vi "GLOBAL CHECKER (PC).vi"() -> ()   [LabVIEW 2013]
panel:
  out "Double 2":dbl
  out "Double 1":dbl
  out "Error 2":bool
  out "Error 1":bool
  # "0.00875"
  # "FF_m of speed controlled by CMD"
  # "-2.5"
  # "FF_b of speed controlled by CMD"
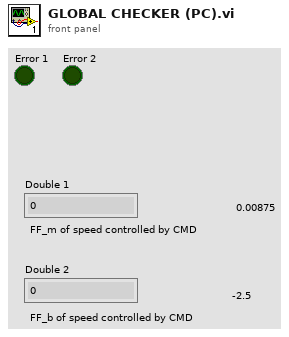
[diagram p1: front panel]
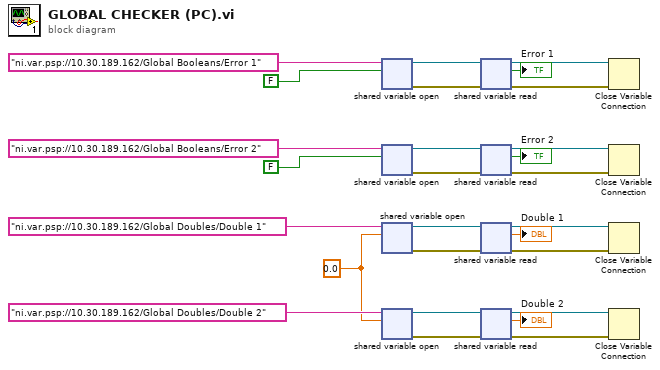
[diagram p0: block diagram]
diagram:
  w3 = 0.0
  n1 = shared-variable-open("ni.var.psp://10.30.189.162/Global Booleans/Error 1", FALSE) -> (w25:refnum<k21>, w22:errorcluster)  [unwired: 2 in]
  n2 = shared-variable-open("ni.var.psp://10.30.189.162/Global Booleans/Error 2", FALSE) -> (w18:refnum<k21>, w21:errorcluster)  [unwired: 2 in]
  n3 = shared-variable-open("ni.var.psp://10.30.189.162/Global Doubles/Double 1", w3) -> (w5:refnum<k21>, w8:errorcluster)  [unwired: 2 in]
  n4 = shared-variable-open("ni.var.psp://10.30.189.162/Global Doubles/Double 2", w3) -> (w12:refnum<k21>, w9:errorcluster)  [unwired: 2 in]
  n5 = shared-variable-read(w25, w22) -> (w24:refnum<k21>, w23:errorcluster, →"Error 1":bool)  [unwired: 1 out]
  n6 = shared-variable-read(w18, w21) -> (w19:refnum<k21>, w20:errorcluster, →"Error 2":bool)  [unwired: 1 out]
  n7 = shared-variable-read(w5, w8) -> (w6:refnum<k21>, w7:errorcluster, →"Double 1":dbl)  [unwired: 1 out]
  n8 = shared-variable-read(w12, w9) -> (w11:refnum<k21>, w10:errorcluster, →"Double 2":dbl)  [unwired: 1 out]
  n9 = Close Variable Connection(8:w23, 11:w24) -> ()  [unwired: 1 out]
  n10 = Close Variable Connection(8:w20, 11:w19) -> ()  [unwired: 1 out]
  n11 = Close Variable Connection(8:w7, 11:w6) -> ()  [unwired: 1 out]
  n12 = Close Variable Connection(8:w10, 11:w11) -> ()  [unwired: 1 out]
